vi "Identify Module Size.vi"(9 "Mod Size Idxs in":T12, 10 "Idx":i32, 11 "RSI Module":T1 {"Module Config Data"."Config Block Data Refs"."Data Reference" format="%.0x"; "CDOutput Data"."BD Refs"."Data Reference" format="%.0x"; "CDInput Data"."BD Refs"."Data Reference" format="%.0x"; "VS ref" format="%.0x"}) -> (1 "Mod Size Idxs out":T12)   [LabVIEW 2016, in "Scan Engine Custom Device.lvlib"]
uses:
  Scan Engine Custom Device.lvlib
  <resource>/objmgr/cRIO.rc
  Type Defs/Mod Size Indexes.ctl
  <vilib>/NI Veristand/Custom Device API/Custom Device Item Ref.ctl
  <vilib>/NI Veristand/Custom Device API/Custom Device API.lvlib
  <vilib>/NI Veristand/Custom Device API/Data Reference.ctl
  <vilib>/NI Veristand/Custom Device API/Block Data Reference.ctl
  Type Defs/Input Data.ctl
  Type Defs/Output Data.ctl
  Modules.lvlibp/RSI Module/Channel Type.ctl
  Modules.lvlibp/RSI Module/RSI Module.lvclass
  Modules.lvlibp/RSI Module/Module Models.ctl
  Type Defs/Module Config Data.ctl
  Type Defs/Mixed IO.ctl
  Type Defs/Open Module IOVs.ctl
  Type Defs/RSI Module Data.ctl
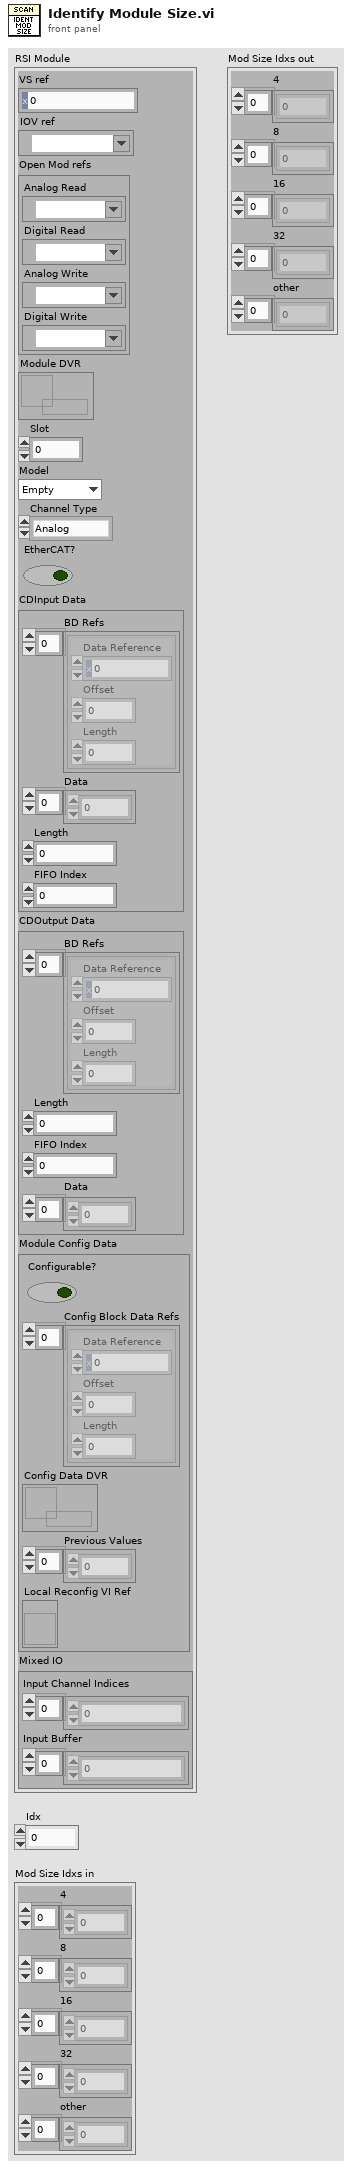
[diagram p1: front panel]
types:
  T1 = typedef "Scan Engine Custom Device.lvlib/RSI Module Data.ctl" = cluster{"VS ref":T2, "IOV ref":refnum<k21>, "Open Mod refs":T3, "Module DVR":refnum<data-value>, "Slot":u32, "Model":T4, "Channel Type":T5, "EtherCAT?":bool, "CDInput Data":T6, "CDOutput Data":T9, "Module Config Data":T10, "Mixed IO":T11}
  T2 = typedef "Custom Device API.lvlib/Custom Device Item Ref.ctl" = u64
  T3 = typedef "Scan Engine Custom Device.lvlib/Open Module IOVs.ctl" = cluster{"Analog Read":refnum<k21>, "Digital Read":refnum<k21>, "Analog Write":refnum<k21>, "Digital Write":refnum<k21>}
  T4 = typedef "Modules.lvlibp/RSI Module.lvclass/Module Models.ctl" = enum16{"Empty", "NI 9201", "NI 9203", "NI 9205", "NI 9206", "NI 9207", "NI 9208", "NI 9211", "NI 9213", "NI 9214", "NI 9215", "NI 9217", "NI 9219", "NI 9221", "NI 9225", "NI 9227", "NI 9229", "NI 9233", "NI 9234", "NI 9235", "NI 9236", "NI 9237", "NI 9239", "NI 9263", "NI 9264", "NI 9265", "NI 9269", "NI 9375", "NI 9401", "NI 9402", "NI 9403", "NI 9411", "NI 9421", "NI 9422", "NI 9423", "NI 9425", "NI 9426", "NI 9435", "NI 9472", "NI 9474", "NI 9475", "NI 9476", "NI 9477", "NI 9478", "NI 9481", "NI 9482", "NI 9485"}
  T5 = typedef "Modules.lvlibp/RSI Module.lvclass/Channel Type.ctl" = enum16{"Analog", "Digital"}
  T6 = typedef "Scan Engine Custom Device.lvlib/Input Data.ctl" = cluster{"BD Refs":T7[], "Data":dbl[], "Length":i32, "FIFO Index":i32}
  T7 = typedef "Custom Device API.lvlib/Block Data Reference.ctl" = cluster{"Data Reference":T8, "Offset":u64, "Length":u64}
  T8 = typedef "Custom Device API.lvlib/Data Reference.ctl" = i32
  T9 = typedef "Scan Engine Custom Device.lvlib/Output Data.ctl" = cluster{"BD Refs":T7[], "Length":i32, "FIFO Index":i32, "Data":dbl[]}
  T10 = typedef "Scan Engine Custom Device.lvlib/Module Config Data.ctl" = cluster{"Configurable?":bool, "Config Block Data Refs":T7[], "Config Data DVR":refnum<data-value>, "Previous Values":dbl[], "Local Reconfig VI Ref":refnum<vi>}
  T11 = typedef "Scan Engine Custom Device.lvlib/Mixed IO.ctl" = cluster{"Input Channel Indices":i32[], "Input Buffer":dbl[]}
  T12 = typedef "Scan Engine Custom Device.lvlib/Mod Size Indexes.ctl" = cluster{"4":i32[], "8":i32[], "16":i32[], "32":i32[], "other":i32[]}
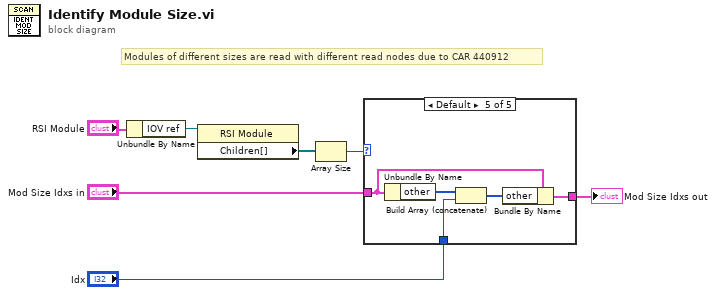
[diagram p0: block diagram]
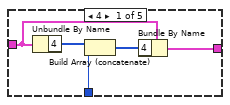
[diagram p2: hidden frame]
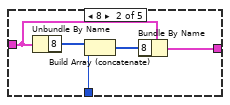
[diagram p3: hidden frame]
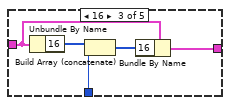
[diagram p4: hidden frame]
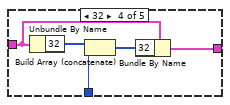
[diagram p5: hidden frame]
diagram:
  # "Modules of different sizes are read with different read nodes due to CAR 440912"
  n1 = Unbundle By Name("RSI Module") -> ("IOV ref"=w2:refnum<k21>)
  n2 = property class="RSI Module"(reference=w2) -> ("Children[]"=w3:refnum<k21>[])  [unwired: 1 in, 2 out]
  n3 = Array Size(array=w3) -> (size(s)=w4:i32)
  n4 = case shown="Default" w4 {
    tunnel: "Mod Size Idxs in" -> [w10 w15 w20 w25 w30]
    tunnel: "Idx" -> [w11 w16 w21 w26 w31]
    tunnel: [w8 w13 w18 w23 w28] -> w7
    frame 4 {
      n5 = Unbundle By Name(w10) -> ("4"=w12:i32[])
      n6 = Build Array (concatenate)(w12, w11) -> (w9:i32[])
      n7 = Bundle By Name(cluster=w10, "4"=w9) -> (w8:T12)
    }
    frame 8 {
      n8 = Unbundle By Name(w15) -> ("8"=w17:i32[])
      n9 = Build Array (concatenate)(w17, w16) -> (w14:i32[])
      n10 = Bundle By Name(cluster=w15, "8"=w14) -> (w13:T12)
    }
    frame 16 {
      n11 = Unbundle By Name(w20) -> ("16"=w22:i32[])
      n12 = Build Array (concatenate)(w22, w21) -> (w19:i32[])
      n13 = Bundle By Name(cluster=w20, "16"=w19) -> (w18:T12)
    }
    frame 32 {
      n14 = Unbundle By Name(w25) -> ("32"=w27:i32[])
      n15 = Build Array (concatenate)(w27, w26) -> (w24:i32[])
      n16 = Bundle By Name(cluster=w25, "32"=w24) -> (w23:T12)
    }
    frame Default {
      n17 = Unbundle By Name(w30) -> ("other"=w32:i32[])
      n18 = Build Array (concatenate)(w32, w31) -> (w29:i32[])
      n19 = Bundle By Name(cluster=w30, "other"=w29) -> (w28:T12)
    }
  }
  "Mod Size Idxs out" <- w7
